vi "pn sequence.vi"() -> ()   [LabVIEW 2014]
panel:
  out "Array":bool[](array[boolean])
  out "Array 5":bool[](array[boolean])
  out "Array 4":bool[](array[boolean])
  out "Array 3":bool[](array[boolean])
  out "Array 2":bool[](array[boolean])
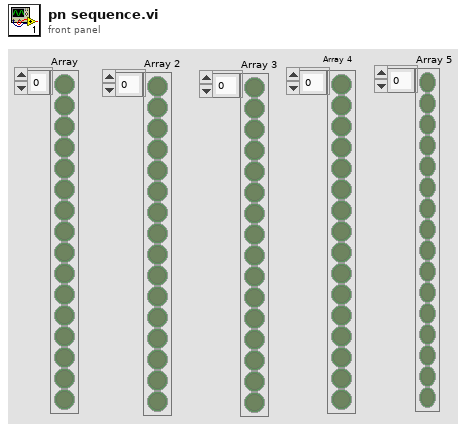
[diagram p1: front panel]
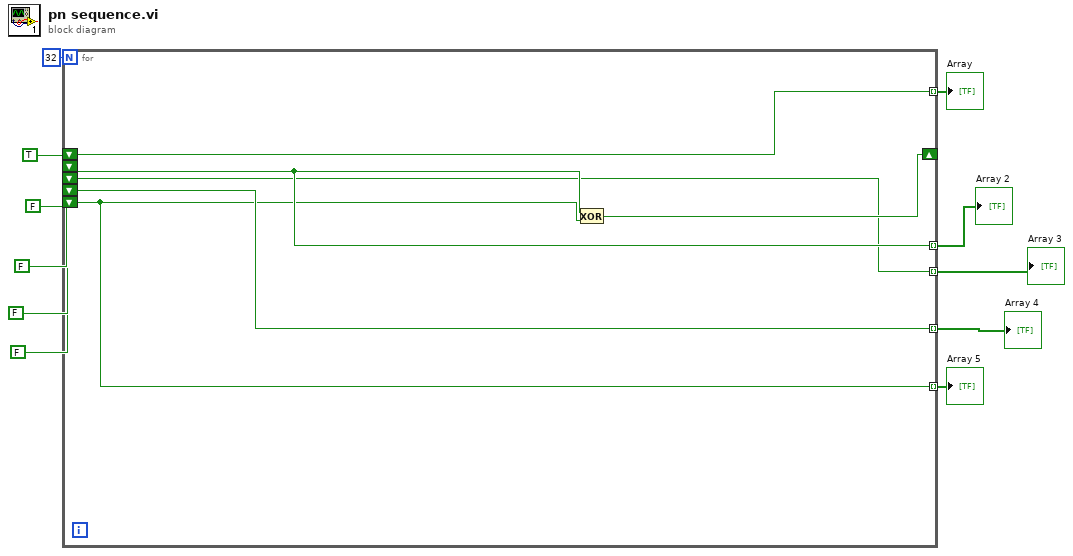
[diagram p0: block diagram]
diagram:
  n1 = for {
    N: 32 -> [_]
    shift-right: [w17] -> _
    shift-left: TRUE -> [w16]
    shift-left: FALSE -> [w15]
    shift-left: FALSE -> [w14]
    shift-left: FALSE -> [w13]
    shift-left: FALSE -> [w12]
    tunnel: [w16] -> w2 mode=indexing
    tunnel: [w15] -> w5 mode=indexing
    tunnel: [w14] -> w4 mode=indexing
    tunnel: [w13] -> w1 mode=indexing
    tunnel: [w12] -> w3 mode=indexing
    n2 = Exclusive Or(1:w12, 2:w15) -> (0:w17:bool)
  }
  "Array 2" <- w5
  "Array 3" <- w4
  "Array 4" <- w1
  "Array 5" <- w3
  "Array" <- w2
